vi "STD溶解氧_获取温度和测量值.vi"(5 "大气压补偿":dbl=1.0, 7 "盐度补偿":dbl, 8 "error in (no error)":errorcluster caption="错误输入（无错误）", 11 "MB session in":refnum<class "MB_Master.lvclass">) -> (0 "error out":errorcluster caption="错误输出", 2 "输出值":cluster{"温度测量值":sgl, "DO%":sgl, "DOmg/L":sgl}, 3 "MB session out":refnum<class "MB_Master.lvclass">)   [LabVIEW 2016, in "斯坦道多参数.lvlib"]
uses:
  <vilib>/Plasmionique/MB Master/MB_Master/MB_Master.lvclass
  <vilib>/Plasmionique/MB Master/MB Master.lvlib
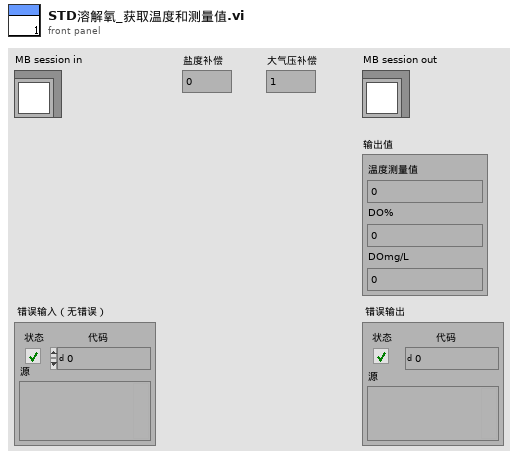
[diagram p1: front panel]
types:
  T1 = cluster{"pH":u32, "DO":u32, "Cond":u32, "Turb":u32, "叶绿素a":u32, "藻密度":u32, "ORP":u32, "COD":u32, "氯化物":u32, "氨氮":u32, "水中油":u32, "悬浮物":u32, "余氯":u32}
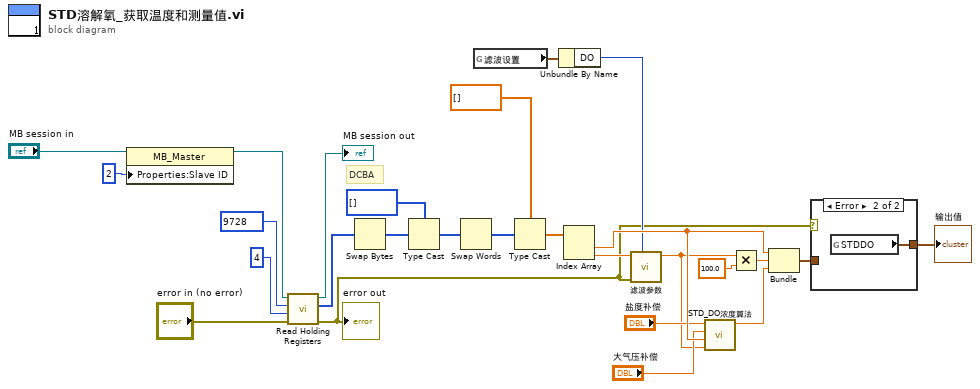
[diagram p0: block diagram]
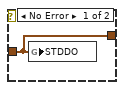
[diagram p2: hidden frame]
diagram:
  # "DCBA"
  n1 = property class="MB_Master"(reference="MB session in", "Properties:Slave ID"=u16 2 ("salve ID")) -> (reference out=w19:refnum<class "MB_Master.lvclass">)  [unwired: 1 in, 1 out]
  n2 = call <vilib>:"Read Holding Registers.vi"("error in (no error)"="error in (no error)", "quantity"=u16 4, "starting address"=u16 9728, "MB session in"=w19) -> ("error out"=w1:errorcluster, "Registers"=w18:u16[], "MB session out"=→"MB session out":refnum<class "MB_Master.lvclass">)  [unwired: 5 in]
  "error out" <- w1
  n3 = Swap Bytes(anything=w18) -> (byte swapped=w17:u16[])
  n4 = Type Cast(type=u32[] [] ("数组 2"), x=w17) -> (*(type *) &x=w23:u32[])
  n5 = Swap Words(1:w23) -> (0:w25:u32[])
  n6 = global read "断电保存变量.vi" "滤波设置"() -> (w5:T1)
  n7 = Type Cast(type=sgl[] [] ("数组 2"), x=w25) -> (*(type *) &x=w21:sgl[])
  n8 = Unbundle By Name(w5) -> ("DO"=w4:u32)
  n9 = Index Array(array=w21) -> (element #1=w16:sgl, element #2=w7:sgl)  [unwired: 2 in]
  n10 = call "滤波参数.vi"("滤波次数"=w4, "error in (no error)"=w1, "x"=w7) -> ("mode"=w6:dbl)  [unwired: 7 in, 1 out]
  n11 = call "STD_DO浓度算法.vi"("溶解氧饱和度值"=w6, "水温"=w16, "大气压补偿"="大气压补偿", "盐度补偿"="盐度补偿") -> ("DataDo_mgL"=w15:dbl)  [unwired: 7 in]
  n12 = Multiply(x=w6, y=sgl 100.0) -> (x*y=w12:dbl)
  n13 = Bundle("数值"=w16, w12, "DataDo_mgL"=w15) -> (w10:cluster{"数值":sgl, dbl, "DataDo_mgL":dbl})  [unwired: 1 in]
  n14 = case shown="Error" w1 {
    tunnel: w10 -> [w28 _]
    tunnel: [w28 w29] -> w3
    frame No Error {
      n15 = global write "禹山过程全局变量.vi" "STDDO"(w28) -> ()
    }
    frame Error {
      n16 = global read "禹山过程全局变量.vi" "STDDO"() -> (w29:cluster{"温度测量值":sgl, "DO%":sgl, "DOmg/L":sgl})
    }
  }
  "输出值" <- w3
